vi "Dialog - Search Sysdef for Custom Devices.vi"(8 "error in (no error)":errorcluster, 10 "CD GUID":string, 11 "Target Node":refnum<k24>) -> (0 "error out":errorcluster, 1 "Custom Device Names":string[](array[string]), 2 "Custom Device Nodes":refnum<k24>[](array[refnum]), 3 "Target Node Out":refnum<k24>)   [LabVIEW 2011]
uses:
  NationalInstruments.VeriStand.SystemStorage
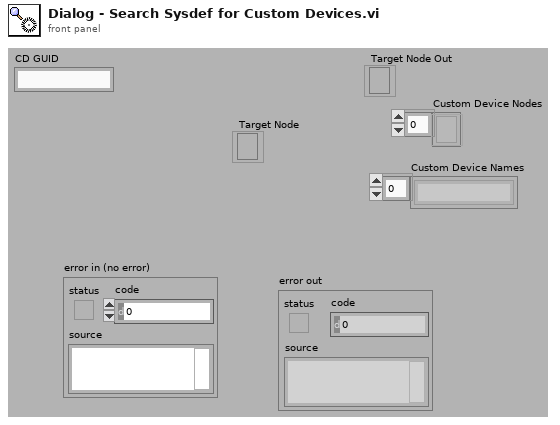
[diagram p1: front panel]
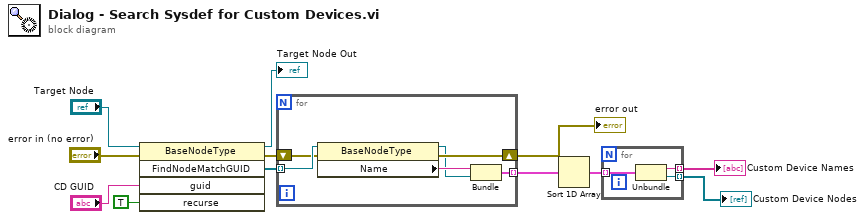
[diagram p0: block diagram]
diagram:
  n1 = invoke class="BaseNodeType" method="FindNodeMatchGUID"(reference="Target Node", error in="error in (no error)", "guid"="CD GUID", "recurse"=TRUE) -> (reference out=→"Target Node Out":refnum<k24>, error out=w11:errorcluster, "FindNodeMatchGUID"=w8:refnum<k24>[])  [unwired: 1 in, 2 out]
  n2 = for {
    tunnel: w8 -> [w18] mode=indexing
    shift-right: [w16] -> w10
    shift-left: w11 -> [w17]
    tunnel: [w15] -> w4 mode=indexing
    n3 = property class="BaseNodeType"(reference=w18, error in=w17) -> (reference out=w13:refnum<k24>, error out=w16:errorcluster, "Name"=w14:string)
    n4 = Bundle("Name"=w14, w13) -> (w15:cluster{"Name":string, refnum<k24>})  [unwired: 1 in]
  }
  "error out" <- w10
  n5 = Sort 1D Array(array=w4) -> (sorted array=w3:cluster{"Name":string, refnum<k24>}[])
  n6 = for {
    tunnel: w3 -> [w21] mode=indexing
    tunnel: [w20] -> w2 mode=indexing
    tunnel: [w19] -> w1 mode=indexing
    n7 = Unbundle(w21) -> ("Name"=w20:string, w19:refnum<k24>)
  }
  "Custom Device Nodes" <- w1
  "Custom Device Names" <- w2
